vi "Práctica9_VISA.vi"() -> ()   [LabVIEW 2018]
uses:
  <vilib>/Instr/_visa.llb/VISA Configure Serial Port (Instr).vi
panel:
  out "read buffer":string
  in  "byte count":u32
  in  "write buffer":string
  in  "VISA resource name":refnum<visa-resource-name>
  out "error out":errorcluster
  # "Anahí Montserrat Vázquez Padilla\nComunicación por VISA\n30/04/2024"
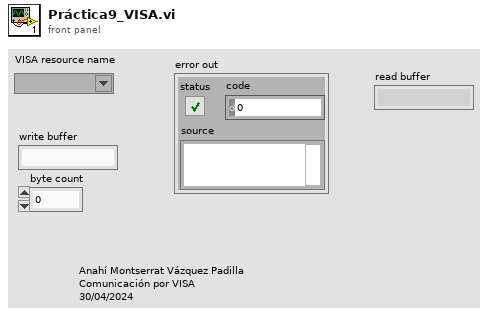
[diagram p1: front panel]
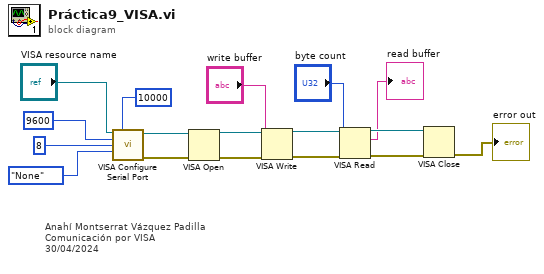
[diagram p0: block diagram]
diagram:
  # "Anahí Montserrat Vázquez Padilla\nComunicación por VISA\n30/04/2024"
  n1 = call-poly "VISA Configure Serial Port"("VISA resource name"="VISA resource name", "timeout (10sec)"=u32 10000, "baud rate (9600)"=9600, "data bits (8)"=8, "parity (0:none)"=enum16{"None", "Odd", "Even", "Mark", "Space"}."None") -> ("VISA resource name out"=w9:refnum<visa-resource-name>, "error out"=w10:errorcluster)  [unwired: 9 in]
  n2 = VISA Open(error in (no error)=w10, VISA resource name=w9) -> (VISA resource name=w16:refnum<visa-resource-name>, error out=w17:errorcluster)  [unwired: 3 in]
  n3 = VISA Write(VISA resource name=w16, write buffer="write buffer", error in (no error)=w17) -> (VISA resource name out=w11:refnum<visa-resource-name>, error out=w15:errorcluster)  [unwired: 1 out]
  n4 = VISA Read(VISA resource name=w11, byte count="byte count", error in (no error)=w15) -> (VISA resource name out=w12:refnum<visa-resource-name>, read buffer=→"read buffer":string, error out=w14:errorcluster)  [unwired: 1 out]
  n5 = VISA Close(VISA resource name=w12, error in (no error)=w14) -> (error out=→"error out":errorcluster)
